vi "Log Result.vi"(8 "error in (no error)":errorcluster, 10 "tdms file":refnum<k34>, 11 "Timestamp Result in":refnum<class "Timestamp Result.lvclass">) -> (0 "error out":errorcluster, 2 "tdms file out":refnum<k34>, 3 "Timestamp Result out":refnum<class "Timestamp Result.lvclass">)   [LabVIEW 2015, in "Timestamp Result.lvclass"]
uses:
  Timestamp Result.lvclass
  Mag Lab Result.lvclass/Mag Lab Result.ctl
  Timestamp Result.lvclass/Timestamp Result.ctl
  Read Group Name.vi
  Read Name.vi
  Read Time Stamp.vi
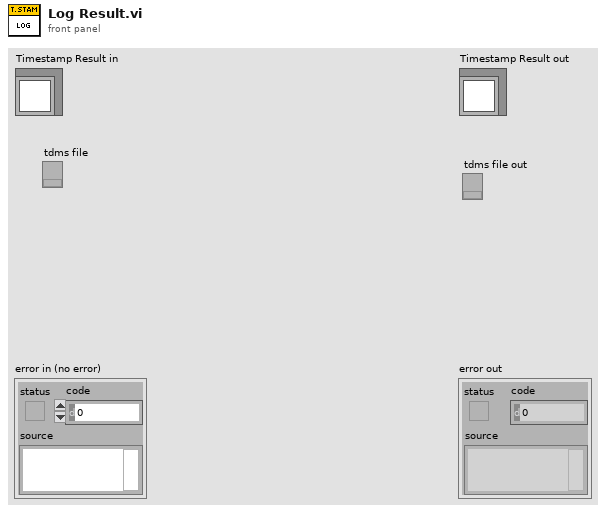
[diagram p1: front panel]
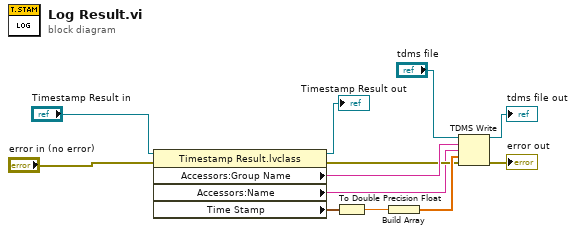
[diagram p0: block diagram]
diagram:
  n1 = property class="Timestamp Result.lvclass"(reference="Timestamp Result in", error in="error in (no error)") -> (reference out=→"Timestamp Result out":refnum<class "Timestamp Result.lvclass">, error out=w3:errorcluster, "Accessors:Group Name"=w5:string, "Accessors:Name"=w1:string, "Time Stamp"=w6:timestamp)
  n2 = To Double Precision Float(number=w6) -> (double precision float=w8:dbl)
  n3 = Build Array(w8) -> (w7:dbl[])
  n4 = TDMS Write(0:"tdms file", 5:w5, 7:w1, 9:w7, 11:w3) -> (4:→"tdms file out":refnum<k34>, 15:→"error out":errorcluster)  [unwired: 1 in, 2 out]
